vi "saveAsDocument.vi"(8 "error in (no error)":errorcluster, 10 "File Path":path, 11 "Document in":refnum<class "Document.lvclass">) -> (0 "error out":errorcluster, 3 "Document out":refnum<class "Document.lvclass">)   [LabVIEW 2020, in "LabVIEW NPOI.lvlib" / "Document.lvclass"]
doc: "Protected dynamic dispatch method to save the <b>Document</b> to the given <b>File Path</b>."
uses:
  Document.lvclass
  D:/Benjamin/Documents/Perso/Code/WC/LabVIEW_NPOI/lib/NPOI 2.1.1/NPOI.OOXML.dll
  lib/NPOI 2.1.1/NPOI.OOXML.dll
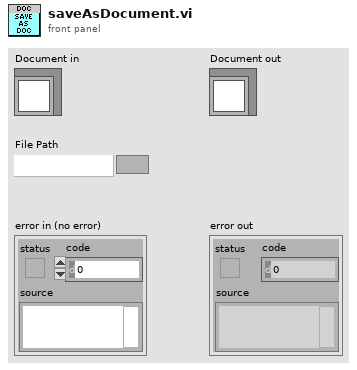
[diagram p1: front panel]
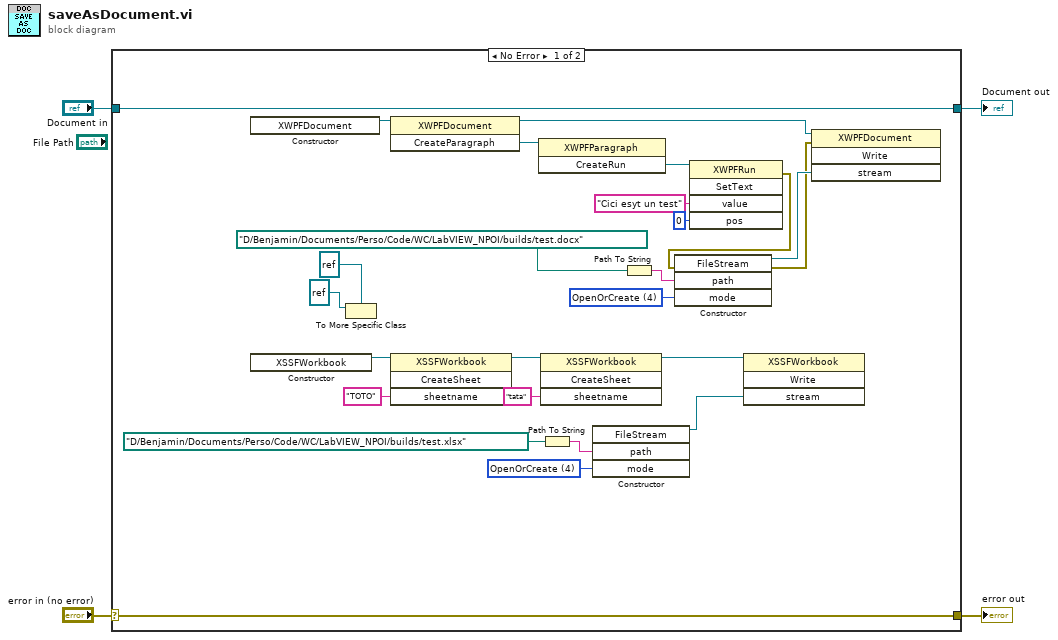
[diagram p0: block diagram]
diagram:
  n1 = case shown="No Error" "error in (no error)" {
    selector: "error in (no error)" -> [w28 w31]
    tunnel: [w28 w31] -> w3
    tunnel: [w29 w30] -> w1
    tunnel: "Document in" -> [w29 w30]
    frame No Error {
      w10 = 4 items=["CreateNew"=1, "Create"=2, "Open"=3, "OpenOrCreate"=4, "Truncate"=5, "Append"=6] ("mode")
      w20 = 4 items=["CreateNew"=1, "Create"=2, "Open"=3, "OpenOrCreate"=4, "Truncate"=5, "Append"=6] ("mode")
      n2 = constructor class="XWPFDocument"() -> (reference out=w27:refnum<k24>)  [unwired: 3 in, 2 out]
      n3 = constructor class="XSSFWorkbook"() -> (reference out=w15:refnum<k24>)  [unwired: 3 in, 2 out]
      n4 = To More Specific Class(target class=refnum<k24> refnum, reference=refnum<k24> refnum ("new reference")) -> ()  [unwired: 1 in, 2 out]
      n5 = invoke class="XWPFDocument" method="CreateParagraph"(reference=w27) -> (reference out=w22:refnum<k24>, "CreateParagraph"=w26:refnum<k24>)  [unwired: 2 in, 1 out]
      n6 = invoke class="XSSFWorkbook" method="CreateSheet"(reference=w15, "sheetname"="TOTO") -> (reference out=w13:refnum<k24>)  [unwired: 2 in, 3 out]
      n7 = invoke class="XWPFParagraph" method="CreateRun"(reference=w26) -> ("CreateRun"=w25:refnum<k24>)  [unwired: 2 in, 2 out]
      n8 = invoke class="XSSFWorkbook" method="CreateSheet"(reference=w13, "sheetname"="tata") -> (reference out=w11:refnum<k24>)  [unwired: 2 in, 3 out]
      n9 = Path To String(path=path "D:/Benjamin/Documents/Perso/Code/WC/LabVIEW_NPOI/builds/test.xlsx") -> (string=w9:string)
      n10 = constructor class="FileStream"("path"=w9, "mode"=w10) -> (reference out=w8:refnum<k24>)  [unwired: 3 in, 4 out]
      n11 = Path To String(path=path "D:/Benjamin/Documents/Perso/Code/WC/LabVIEW_NPOI/builds/test.docx") -> (string=w21:string)
      n12 = invoke class="XWPFRun" method="SetText"(reference=w25, "value"="Cici esyt un test", "pos"=0) -> (error out=w17:errorcluster)  [unwired: 2 in, 4 out]
      n13 = constructor class="FileStream"(error in=w17, "path"=w21, "mode"=w20) -> (reference out=w19:refnum<k24>, error out=w16:errorcluster)  [unwired: 2 in, 3 out]
      n14 = invoke class="XSSFWorkbook" method="Write"(reference=w11, "stream"=w8) -> ()  [unwired: 2 in, 4 out]
      n15 = invoke class="XWPFDocument" method="Write"(reference=w22, error in=w16, "stream"=w19) -> ()  [unwired: 1 in, 4 out]
    }
    frame Error {
    }
  }
  "error out" <- w3
  "Document out" <- w1
